vi "线粗.vi"(11 "字符串":string) -> (3 "线粗":u8)   [LabVIEW 2014]
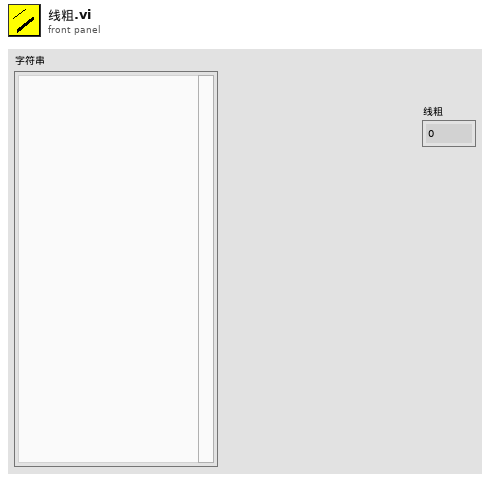
[diagram p1: front panel]
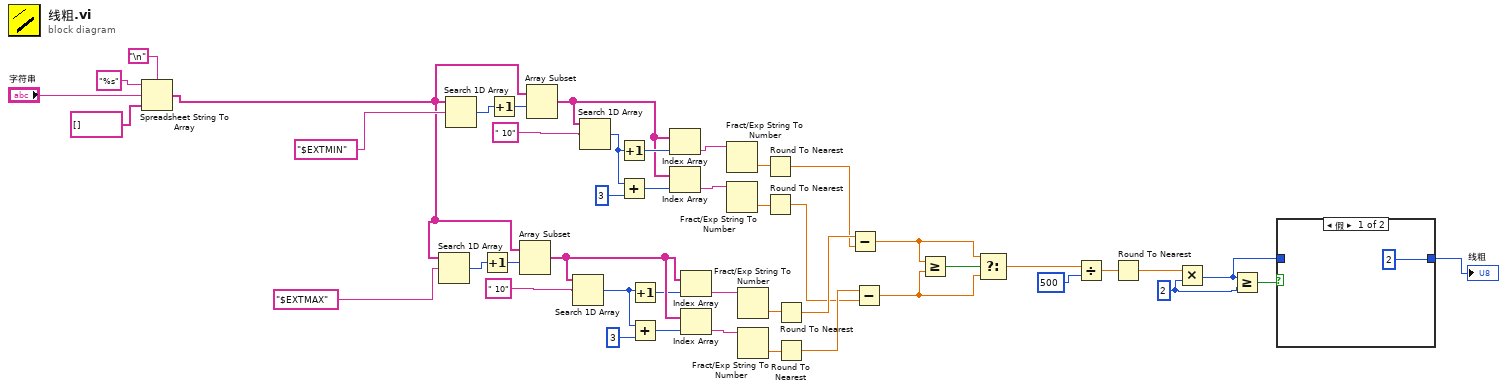
[diagram p0: block diagram]
diagram:
  w4 = u16 2 ("y")
  n1 = Spreadsheet String To Array(delimiter (Tab)="\n", format string="%s" ("格式字符串"), spreadsheet string="字符串", array type (2D Dbl)=string[] [] ("数组类型(2D Dbl)")) -> (array=w5:string[])
  n2 = Search 1D Array(1D array=w5, element="$EXTMAX" ("元素")) -> (index of element=w28:i32)  [unwired: 1 in]
  n3 = Search 1D Array(1D array=w5, element="$EXTMIN" ("元素")) -> (index of element=w40:i32)  [unwired: 1 in]
  n4 = Increment(x=w28) -> (x+1=w27:i32)
  n5 = Increment(x=w40) -> (x+1=w41:i32)
  n6 = Array Subset(array=w5, index=w27) -> (w19:string[])  [unwired: 1 in]
  n7 = Array Subset(array=w5, index=w41) -> (w38:string[])  [unwired: 1 in]
  n8 = Search 1D Array(1D array=w19, element=" 10") -> (index of element=w20:i32)  [unwired: 1 in]
  n9 = Search 1D Array(1D array=w38, element=" 10") -> (index of element=w35:i32)  [unwired: 1 in]
  n10 = Increment(x=w35) -> (x+1=w39:i32)
  n11 = Add(x=w35, y=i8 3) -> (x+y=w37:i32)
  n12 = Increment(x=w20) -> (x+1=w17:i32)
  n13 = Add(x=w20, y=i8 3) -> (x+y=w21:i32)
  n14 = Index Array(array=w38, index=w39) -> (element=w34:string)
  n15 = Index Array(array=w38, index=w37) -> (element=w33:string)
  n16 = Index Array(array=w19, index=w17) -> (element=w18:string)
  n17 = Index Array(array=w19, index=w21) -> (element=w23:string)
  n18 = Fract/Exp String To Number(string=w34) -> (number=w32:dbl)  [unwired: 3 in, 1 out]
  n19 = Fract/Exp String To Number(string=w33) -> (number=w31:dbl)  [unwired: 3 in, 1 out]
  n20 = Fract/Exp String To Number(string=w18) -> (number=w24:dbl)  [unwired: 3 in, 1 out]
  n21 = Fract/Exp String To Number(string=w23) -> (number=w25:dbl)  [unwired: 3 in, 1 out]
  n22 = Round To Nearest(number=w32) -> (nearest integer value=w15:dbl)
  n23 = Round To Nearest(number=w31) -> (nearest integer value=w13:dbl)
  n24 = Round To Nearest(number=w24) -> (nearest integer value=w16:dbl)
  n25 = Round To Nearest(number=w25) -> (nearest integer value=w14:dbl)
  n26 = Subtract(x=w16, y=w15) -> (x-y=w11:dbl)
  n27 = Subtract(x=w14, y=w13) -> (x-y=w10:dbl)
  n28 = Greater Or Equal?(x=w11, y=w10) -> (x >= y?=w12:bool)
  n29 = Select(t=w11, s=w12, f=w10) -> (s? t:f=w8:dbl)
  n30 = Divide(x=w8, y=u16 500) -> (x/y=w7:dbl)
  n31 = Round To Nearest(number=w7) -> (nearest integer value=w6:dbl)
  n32 = Multiply ("乘")(x=w6, y=w4) -> (x*y=w1:u8)
  n33 = Greater Or Equal?(x=w1, y=w4) -> (x >= y?=w3:bool)
  n34 = case shown="假" w3 {
    tunnel: w1 -> [_ w48]
    tunnel: [2 w48] -> w2
    frame False {
    }
    frame True {
    }
  }
  "线粗" <- w2
